vi "Progress Bar.vi"(8 "error in":errorcluster, 10 "N":i32, 11 "i":i32) -> (0 "error out":errorcluster, 2 "Stop?":bool, 3 "Progress Bar":u8(slide) caption="Analysis Complete" scale=0.0..100.0)   [LabVIEW 2024]
panel:
  in  "Stop":bool
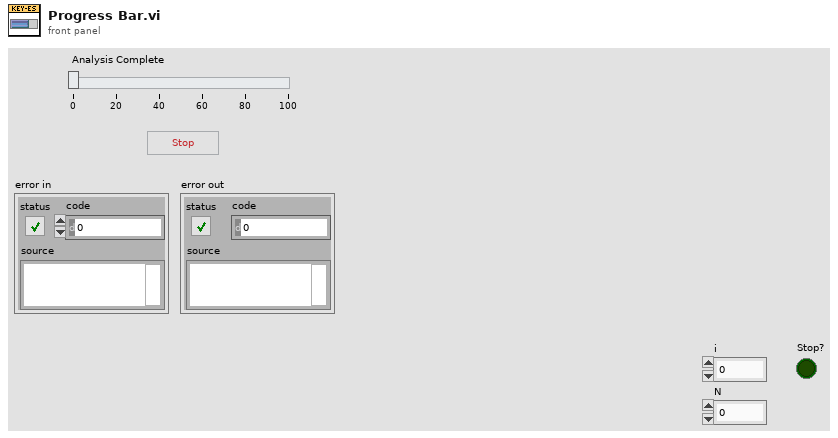
[diagram p1: front panel]
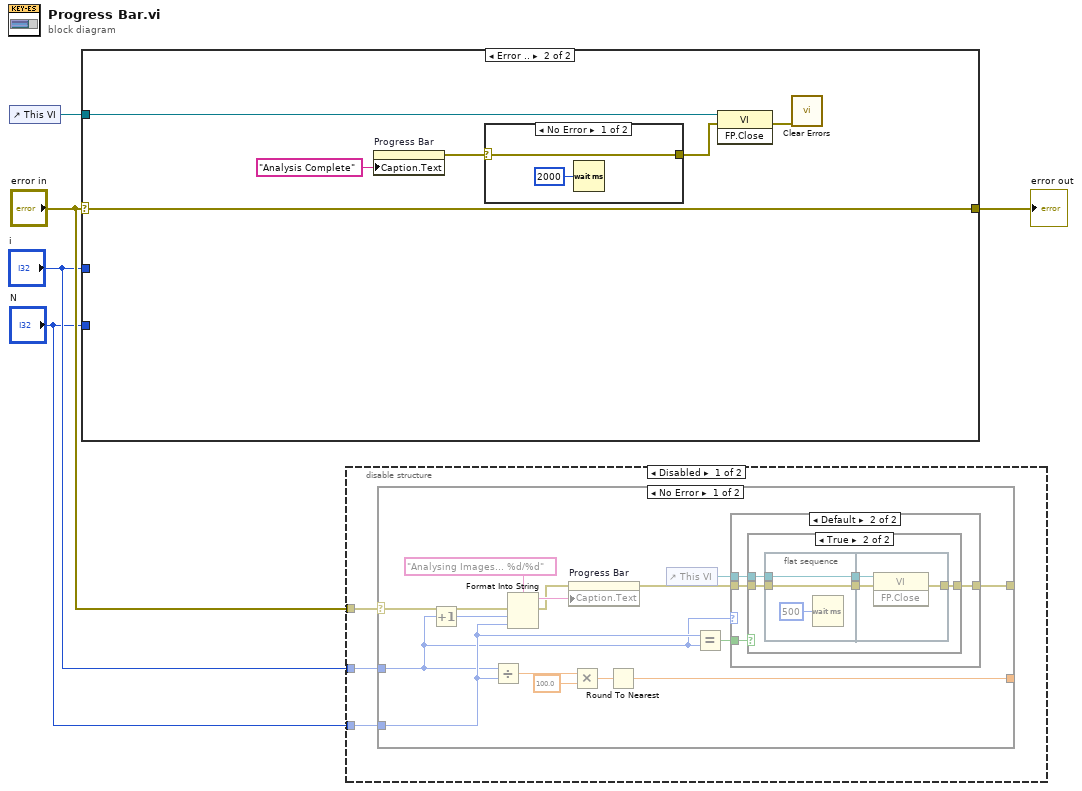
[diagram p0: block diagram]
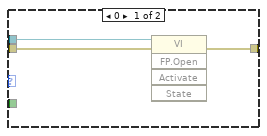
[diagram p2: hidden frame]
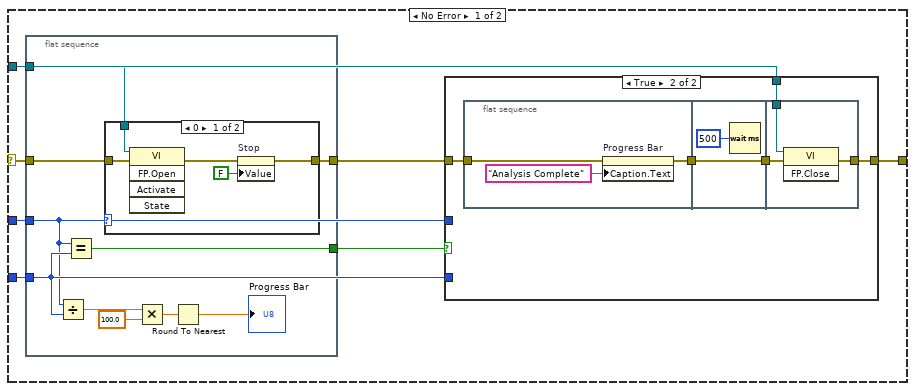
[diagram p6: hidden frame]
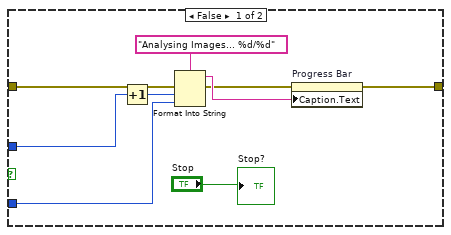
[diagram p8: hidden frame]
diagram:
  n1 = control-ref of="This VI"() -> (w1:refnum<vi>)
  n2 = case shown="Error .." "error in" {
    selector: "error in" -> [w8 w56]
    tunnel: "i" -> [w6 _]
    tunnel: "N" -> [w10 _]
    tunnel: [w12 w56] -> w5
    tunnel: w1 -> [w7 w55]
    frame No Error {
      n3 = flat-sequence {
        tunnel: w10 -> [w18]
        tunnel: w8 -> [w17]
        tunnel: w7 -> [w16]
        tunnel: w6 -> [w15]
        tunnel: [w22] -> w11
        tunnel: [w13] -> w9
        frame #0 {
          n4 = Divide(x=w15, y=w18) -> (x/y=w21:dbl)
          n5 = Equal?(x=w15, y=w18) -> (x = y?=w22:bool)
          n6 = case shown="0" w15 {
            tunnel: [w24 w28] -> w13
            tunnel: w17 -> [w27 w28]
            tunnel: w16 -> [w26 _]
            frame 0 {
              n7 = invoke class="VI" method="FP.Open"(reference=w26, error in=w27) -> (error out=w23:errorcluster)  [unwired: 3 in, 4 out]
              n8 = property on="Stop" class="Bool (strict)"(error in=w23, "Value"=FALSE ("Stop")) -> (error out=w24:errorcluster)  [unwired: 1 in, 1 out]
            }
            frame Default {
            }
          }
          n9 = Multiply(x=w21, y=100.0) -> (x*y=w19:dbl)
          n10 = Round To Nearest(number=w19) -> (nearest integer value=→"Progress Bar":dbl)
        }
      }
      n11 = case shown="True" w11 {
        tunnel: w9 -> [w34 w41]
        tunnel: [w30 w42] -> w12
        tunnel: w10 -> [w33 _]
        tunnel: w6 -> [w32 _]
        tunnel: w7 -> [_ w40]
        frame False {
          n12 = Increment(x=w32) -> (x+1=w31:i32)
          n13 = Format Into String(format string="Analysing Images... %d/%d", error in=w34, w31, w33) -> (resulting string=w36:string, error out=w35:errorcluster)  [unwired: 1 in]
          n14 = property on="Progress Bar" class="Slide (strict)"(error in=w35, "Caption.Text"=w36) -> (error out=w30:errorcluster)  [unwired: 1 in, 1 out]
          "Stop?" <- "Stop"
        }
        frame True {
          n15 = flat-sequence {
            tunnel: w41 -> [w44]
            tunnel: [w43] -> w39
            tunnel: w39 -> [w47]
            tunnel: [w47] -> w38
            tunnel: [w50] -> w42
            tunnel: w38 -> [w49]
            tunnel: w40 -> [w48]
            frame #0 {
              n16 = property on="Progress Bar" class="Slide (strict)"(error in=w44, "Caption.Text"="Analysis Complete") -> (error out=w43:errorcluster)  [unwired: 1 in, 1 out]
            }
            frame #1 {
              n17 = Wait (ms)(milliseconds to wait=u32 500) -> ()  [unwired: 1 out]
            }
            frame #2 {
              n18 = invoke class="VI" method="FP.Close"(reference=w48, error in=w49) -> (error out=w50:errorcluster)  [unwired: 1 in, 2 out]
            }
          }
        }
      }
    }
    frame Error {
      n19 = property on="Progress Bar" class="Slide (strict)"("Caption.Text"="Analysis Complete") -> (error out=w53:errorcluster)  [unwired: 2 in, 1 out]
      n20 = case shown="No Error" w53 {
        selector: w53 -> [w58 w59]
        tunnel: [w58 w59] -> w52
        frame No Error {
          n21 = Wait (ms)(milliseconds to wait=u32 2000) -> ()  [unwired: 1 out]
        }
        frame Error {
        }
      }
      n22 = invoke class="VI" method="FP.Close"(reference=w55, error in=w52) -> (error out=w51:errorcluster)  [unwired: 1 in, 2 out]
      n23 = call <vilib>:"Clear Errors.vi"("error in (no error)"=w51) -> ()  [unwired: 5 in, 2 out]
    }
  }
  "error out" <- w5
  n24 = disable-structure shown="Disabled" {
    disable-tunnel: "error in" -> [w62 _]
    disable-tunnel: "i" -> [w61 _]
    disable-tunnel: "N" -> [w60 _]
    frame Disabled {
      n25 = case shown="No Error" w62 {
        selector: w62 -> [w70 w97]
        tunnel: [w74 _] -> _
        tunnel: w61 -> [w64 _]
        tunnel: w60 -> [w66 _]
        tunnel: [w67 w97] -> _
        frame No Error {
          n26 = Increment(x=w64) -> (x+1=w63:i32)
          n27 = Divide(x=w64, y=w66) -> (x/y=w77:dbl)
          n28 = Format Into String(format string="Analysing Images... %d/%d", error in=w70, w63, w66) -> (resulting string=w72:string, error out=w71:errorcluster)  [unwired: 1 in]
          n29 = property on="Progress Bar" class="Slide (strict)"(error in=w71, "Caption.Text"=w72) -> (error out=w68:errorcluster)  [unwired: 1 in, 1 out]
          n30 = Multiply(x=w77, y=100.0) -> (x*y=w75:dbl)
          n31 = Round To Nearest(number=w75) -> (nearest integer value=w74:dbl)
          n32 = control-ref of="This VI"() -> (w69:refnum<vi>)
          n33 = Equal?(x=w66, y=w64) -> (x = y?=w65:bool)
          n34 = case shown="Default" w64 {
            tunnel: w69 -> [w80 w84]
            tunnel: [w78 w83] -> w67
            tunnel: w68 -> [w79 w82]
            tunnel: w65 -> [_ w81]
            frame 0 {
              n35 = invoke class="VI" method="FP.Open"(reference=w80, error in=w79) -> (error out=w78:errorcluster)  [unwired: 3 in, 4 out]
            }
            frame Default {
              n36 = case shown="True" w81 {
                tunnel: w84 -> [_ w88]
                tunnel: [w85 w87] -> w83
                tunnel: w82 -> [w85 w86]
                frame False {
                }
                frame True {
                  n37 = flat-sequence {
                    tunnel: w88 -> [w93]
                    tunnel: [w93] -> w90
                    tunnel: w86 -> [w91]
                    tunnel: [w91] -> w89
                    tunnel: w90 -> [w96]
                    tunnel: [w95] -> w87
                    tunnel: w89 -> [w94]
                    frame #0 {
                      n38 = Wait (ms)(milliseconds to wait=u32 500) -> ()  [unwired: 1 out]
                    }
                    frame #1 {
                      n39 = invoke class="VI" method="FP.Close"(reference=w96, error in=w94) -> (error out=w95:errorcluster)  [unwired: 1 in, 2 out]
                    }
                  }
                }
              }
            }
          }
        }
        frame Error {
        }
      }
    }
    frame Enabled {
    }
  }
